vi "Roller Loop.vi"   [LabVIEW 2015]
uses:
  Common Code/Roller Indicators.ctl
  Common Code/Roller Mode Enum.ctl
  Common Code/Auto Roller Commands.ctl
  Common Code/Inner Roller States.ctl
  Sensors/Pot Data.ctl
  Untip Can States.ctl
  Roller Modes.ctl
  Really Real Manual Align.ctl
  Common Code/Change Detect Int.vi
  Robot Global Data.vi
  <vilib>/Rock Robotics/WPI/Solenoid/Deprecated/WPI_SolenoidSetBool.vi
types:
  T1 = typedef "Roller Modes.ctl" = cluster{"Auto Roller Command":T2, "Roller Mode":T3, "Override Intake Speed":dbl}
  T2 = typedef "Auto Roller Commands.ctl" = enum16{"Drag Tote", "Grab Tote", "Idle", "Eject Tote", "Untip Can", "Grab Can"}
  T3 = typedef "Roller Mode Enum.ctl" = enum16{"Manual", "Safe", "Auto"}
  T4 = typedef "Inner Roller States.ctl" = enum16{"Turn Tote Portrait", "Acquire Tote", "Absorb Tote", "Turn Tote Right", "Turn Tote Left", "Acquire Can", "Absorb Can", "Turn Can", "Hold Tote"}
  T5 = typedef "Roller Indicators.ctl" = cluster{"Rollers Closed?":bool, "Roller Mode":T3, "Auto Roller State":T2, "Tote Inside?":bool, "Intake State":T4, "Left Ping Dist":sgl, "Right Ping Dist":sgl, "Potentiometer Cluster":T6, "PING Decision":T4, "Left Arm Closed?":bool, "Portrait?":bool, "Right Arm Closed?":bool, "Left Out":sgl, "Right Out":sgl, "Left Current":sgl, "Right Current":sgl, "Tote Load Complete?":bool, "Untip Complete?":bool, "Untip State":T7, "Roller Safety Open":bool}
  T6 = typedef "Pot Data.ctl" = cluster{"Left Pot Zero":sgl, "Right Pot Zero":sgl, "Left Potentiometer":sgl, "Right Potentiometer":sgl, "Left Pot Non Zero":sgl, "Right Pot Non Zero":sgl}
  T7 = typedef "Untip Can States.ctl" = enum16{"Release Can", "Catch Can", "Idle"}
  T8 = typedef "Dashboard Control Data.ctl" = cluster{"Cam Exposure":dbl, "Go to angle":dbl, "Steer PID Gains":cluster{"proportional gain (Kc)":dbl, "integral time (Ti, min)":dbl, "derivative time (Td, min)":dbl}, "Steer PID output Range":cluster{"output high":dbl, "output low":dbl}, "Pressure m \nValue":dbl, "Pressure b \nValue":dbl, "Roller Command Cluster ":T9, "Elevator":T10, "Encoder Control":T12, "Auton Settings":cluster{"Drive Dist Window Size":dbl}, "Drivetrain Settings":T13, "Lance":T14}
  T9 = typedef "Roller Control.ctl" = cluster{"Intake Speed":dbl, "Turn In Speed":dbl, "Unload Speed":dbl, "Turn Out Speed":dbl, "Ping Align Tolerance":dbl, "Tote Range Threshold":dbl, "Right Pot 0":dbl, "Pot Threshold":dbl, "Left Pot 0":dbl, "Right Pot Scale":dbl, "Left Pot Scale":dbl, "Min Elevator Height":dbl, "Eject Time":dbl, "Eject US Threshold":dbl, "Anti-Twitch Time":u32, "Ping Caring Threshold":dbl, "Pot Diff Threshold":dbl, "Pinch Sustain":u32, "Absorb Give Up Threshold":dbl, "Untip In Threshold":dbl, "Untip Grab Range":dbl, "Ultrasonic Hold Time":u32, "Landscape Absorb Time":u32, "Pot Use Wait Time":u32, "Can Turn Stop Range":dbl, "HP Load Speed":dbl, "Stick Multiplier":dbl, "Coop Eject Speed":dbl}
  T10 = typedef "Elevator DB Control.ctl" = cluster{"PID Output Range":cluster{"output high":dbl, "output low":dbl}, "PID gains":cluster{"proportional gain (Kc)":dbl, "integral time (Ti, min)":dbl, "derivative time (Td, min)":dbl}, "Height Tolerance":sgl, " Encoder Constant":dbl, "Eject Time":sgl, "Zeroing Speed":sgl, "Presets":T11, "Ping Detect Threshold":sgl, "Trashcan Detect Threshold":sgl, "Zero Filter Time":dbl, "Stabilizer Open Time":dbl, "Zero Creep Speed":dbl, "Max Current":dbl, "Current Trip Time":dbl, "Abort Pitch":dbl, "Finger m":dbl, "Finger b":dbl, "Finger max ":dbl, "Finger Stabilizer":dbl, "Finger Store":dbl, "Finger Stop Store":dbl, "Stabilizer Close Time":dbl, "Finger min":dbl, "Unstick gain":dbl, "Full Detect Max":dbl}
  T11 = typedef "Elevator Presets.ctl" = cluster{"Pickup 2 w/ Tote":sgl, "Pickup 2 w/ Trashcan":sgl, "Pickup 3 w/ Tote":sgl, "Pickup 3 w/ Trashcan":sgl, "Bottom":sgl, "Pickup 1 w/ Tote":sgl, "Pickup Trashcan":sgl, "Pickup 1 w/ Trashcan":sgl, "Eject":sgl, "Hold Low":sgl, "Step add height":sgl, "Untip Lift":dbl, "Drop Stack":dbl, "HP Load Hold":dbl, "HP Load Drop":dbl, "HP Load Hold Can":dbl, "Store can max":dbl, "HP Drag Score":dbl, "HP Drag Finish":dbl, "Finger trashcan avoid":dbl, "Full":dbl}
  T12 = typedef "Encoder Control.ctl" = cluster{"Left Tick Constant":dbl, "Right Tick Constant":dbl, "Center Tick Constant":dbl, "Reset?":bool, "Y Dist":cluster{"PID gains":cluster{"proportional gain (Kc)":dbl, "integral time (Ti, min)":dbl, "derivative time (Td, min)":dbl}}, "X Dist":cluster{"PID gains":cluster{"proportional gain (Kc)":dbl, "integral time (Ti, min)":dbl, "derivative time (Td, min)":dbl}}, "Y Stop Thresh":dbl, "Y Stop Speed":dbl, "X Stop Thresh":dbl, "X Stop Speed":dbl}
  T13 = typedef "Drivetrain Settings.ctl" = cluster{"Gyro Tolerance":sgl, "Strafe Correct max steer":sgl, "Strafe Timer Wait":sgl, "Throttle Ramp (ms)":sgl, "Strafe Ramp (ms)":sgl, "Angular rate compensation":bool, "Throttle to Rate Scale":sgl, "Rate compensation gain":sgl, "Creep Steer":sgl, "Creep Throttle":sgl}
  T14 = typedef "Pike DB Controls.ctl" = cluster{"Down Speed":dbl, "Up Speed":dbl, "Max Down Time":dbl, "Max Up Time":dbl, "Current Limit":dbl}
  T15 = typedef "Ultrasonic Indicators.ctl" = cluster{"Left Distance":dbl, "Right Distance":dbl, "Center Distance":dbl, "Left Distance Unfilter":dbl, "Right Distance Unfilter":dbl, "Center Distance Unfilter":dbl}
  T16 = typedef "Roller Manual Bools.ctl" = cluster{"Manual Claw":bool, "Manual Align":T17, "Left Speed":dbl, "Right Speed":dbl}
  T17 = typedef "Really Real Manual Align.ctl" = enum16{"In", "Left", "Right", "Out", "Idle", "HP Load", "Speeds"}
  T18 = typedef "Elevator Status.ctl" = cluster{"Height":dbl, "Enc Value":dbl, "Limit Override":bool, "Mode":T19, "High IR":bool, "Motor Out":dbl, "Ping Detect":bool, "Auto Elevator Indicators":T20, "Master Current":dbl, "Slave Current":dbl, "High Current":bool, "Current Tripped":bool, "Top Limit":bool, "Bottom Limit":bool, "Eject Piston":bool, "Stabilizer":bool, "Finger":bool, "Finger Height":dbl, "Finger Raw":dbl, "Finger at Bottom":bool}
  T19 = typedef "Elevator Mode.ctl" = enum16{"Manual", "Safe", "Auto"}
  T20 = typedef "Auto Elevator Indicators.ctl" = cluster{"Target Out":dbl, "Storing Trashcan?":bool, "State":T21, "In Range":bool, "Store Can Command":bool, "HP Load":bool}
  T21 = typedef "Elevator State.ctl" = enum16{"Idle", "Goto Load Position", "Wait for Load", "Load Drop", "Load Lift", "Drop Stack", "Goto Eject Position", "Eject ", "Raise Trashcan", "Open Stabilizer", "Untip Drop", "Untip Wait", "Untip Lift", "Abort Load", "HP Load Wait", "HP Load Drop", "HP Load Lift", "HP Load Abort", "Close Stabilizer", "HP Load Unfinish", "HP Load Score", "HP Load Finish", "HP Goto Finish Down", "HP Goto Finish Up", "Full"}
  T22 = typedef "WPI_MotorControlDeviceRef.ctl" = cluster{"DeviceStatus":errorcluster, "Type":T23, "PWM":cluster{"PWM Channel":T24, "DeadBand":T25}, "CAN":cluster{"Device Number":u8, "Control Mode":T26, "Semaphore":T27, "Max Vout":dbl, "TalonSRX Control Mode":T28}, "Invert":bool, "TransformRef":T29, "InvTransformRef":T29}
  T23 = typedef "WPI_MotorControlType.ctl" = enum16{"PWM", "CAN", "CANTalonSRX"}
  T24 = typedef "FPGA_DIOPWMChannel.ctl" = enum8{"PWM 0", "PWM 1", "PWM 2", "PWM 3", "PWM 4", "PWM 5", "PWM 6", "PWM 7", "PWM 8", "PWM 9", "PWM MXP 0", "PWM MXP 1", "PWM MXP 2", "PWM MXP 3", "PWM MXP 4", "PWM MXP 5", "PWM MXP 6", "PWM MXP 7", "PWM MXP 8", "PWM MXP 9", "Invalid"}
  T25 = typedef "WPI_PWMDeadband.ctl" = cluster{"Name":string, "maxPositivePwm":i32, "minPositivePwm":i32, "centerPwm":i32, "maxNegativePwm":i32, "minNegativePwm":i32, "angularRange":u16}
  T26 = typedef "WPI_CANJaguar_ControlMode.ctl" = enum8{"Percent VBus", "Current", "Speed", "Position", "Voltage"}
  T27 = typedef "Semaphore RefNum" = refnum<k1>
  T28 = typedef "WPI_CANTalonSRX_APIControlMode.ctl" = enum8{"Percent VBus", "Speed", "Position", "Slave", "Unchanged / Invalid"}
  T29 = typedef "WPI_PWMTransform_ConPane.ctl" = refnum<vi>
  T30 = typedef "WPI_SolenoidDevRef.ctl" = cluster{"DevStatus":errorcluster, "Pneumatics Control Module":u8, "Forward Solenoid Channel":T31, "Reverse Solenoid Channel":T31}
  T31 = typedef "WPI_SolenoidChannel.ctl" = enum8{"Solenoid 0", "Solenoid 1", "Solenoid 2", "Solenoid 3", "Solenoid 4", "Solenoid 5", "Solenoid 6", "Solenoid 7", "Invalid"}
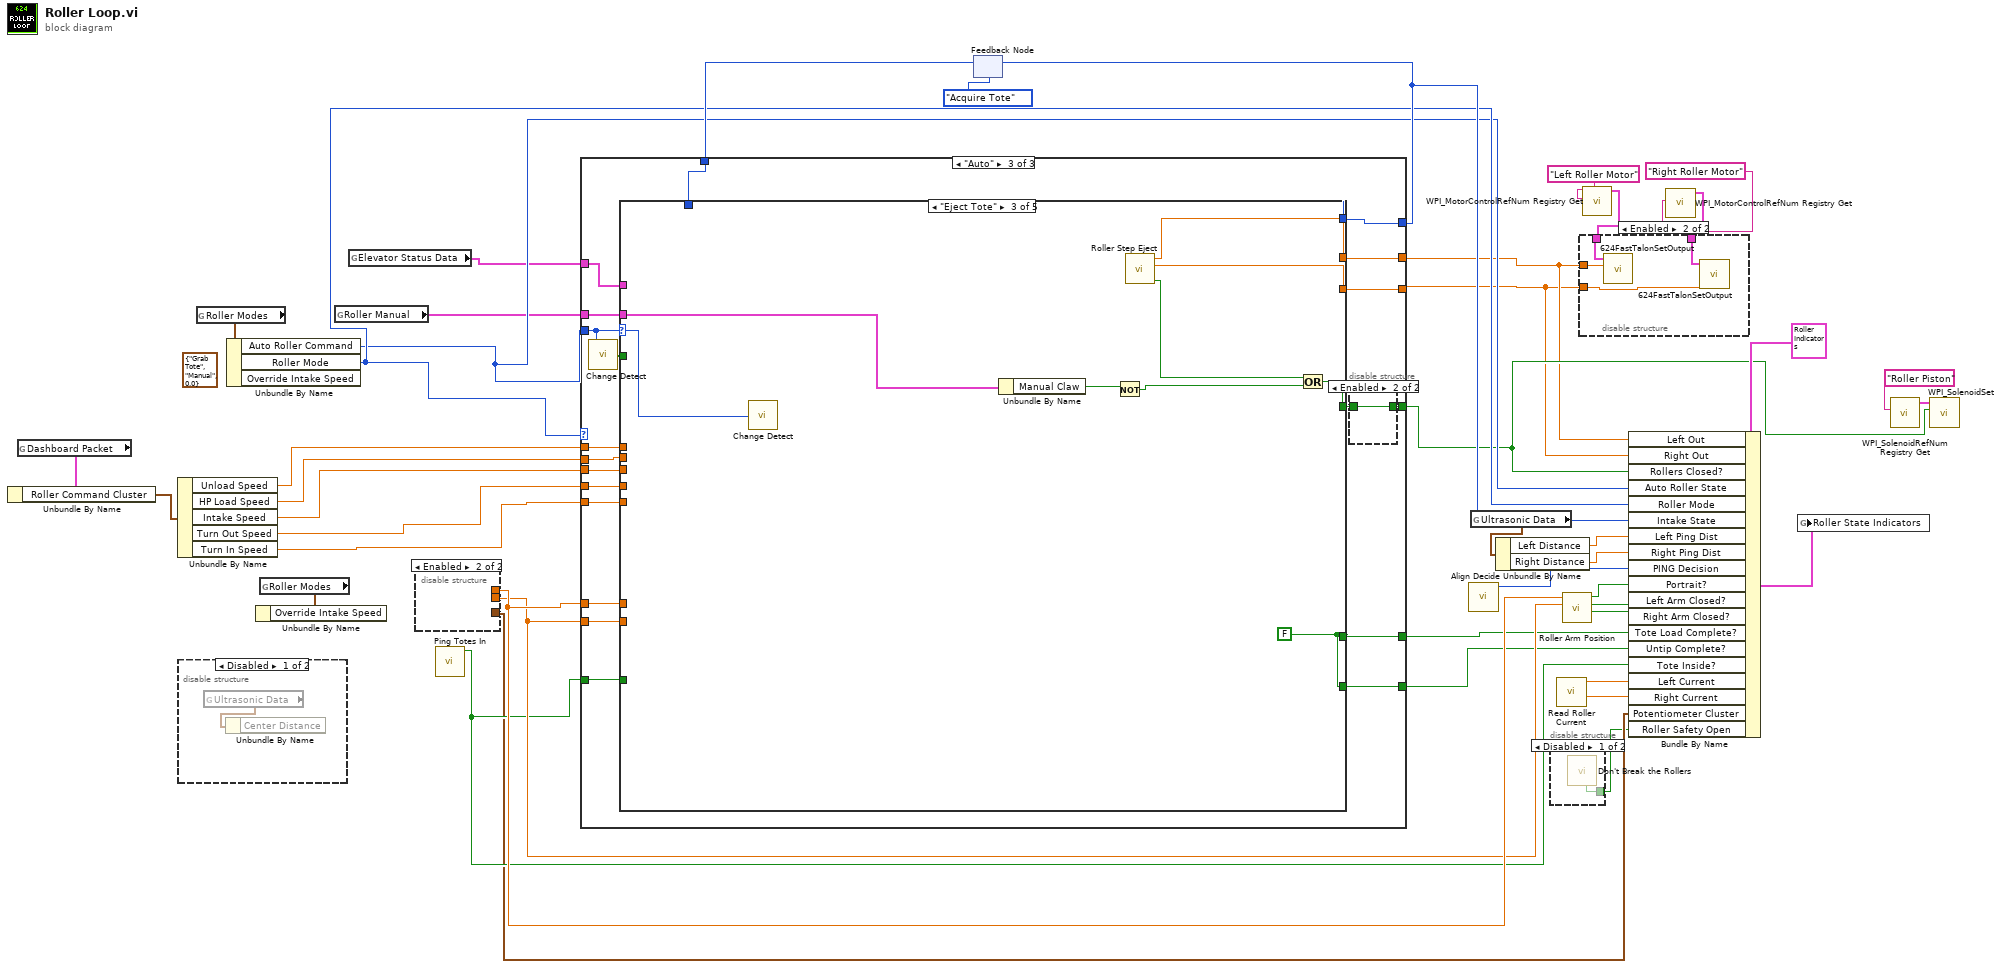
[diagram p0: block diagram]
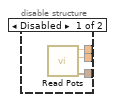
[diagram p2: hidden frame]
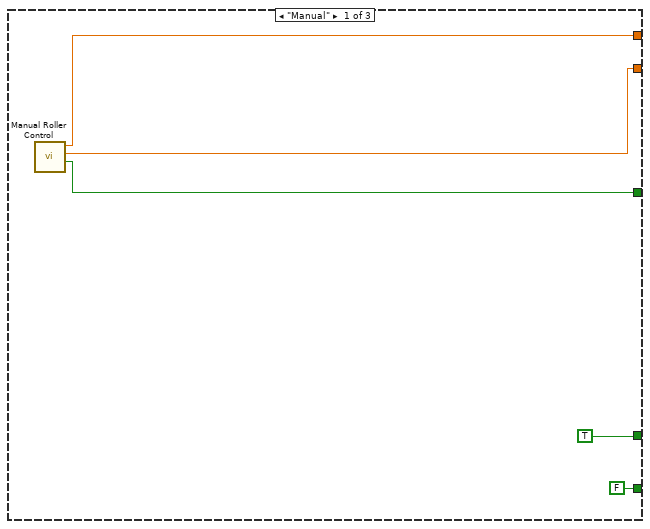
[diagram p4: hidden frame]
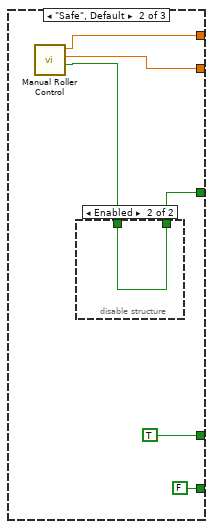
[diagram p5: hidden frame]
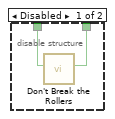
[diagram p6: hidden frame]
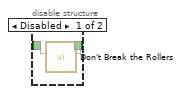
[diagram p7: hidden frame]
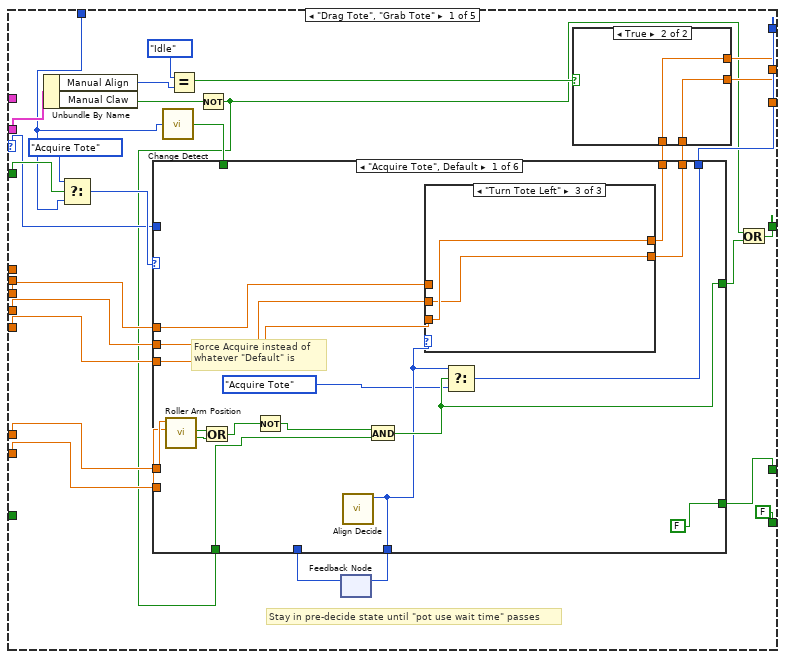
[diagram p8: hidden frame]
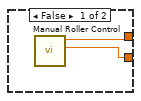
[diagram p9: hidden frame]
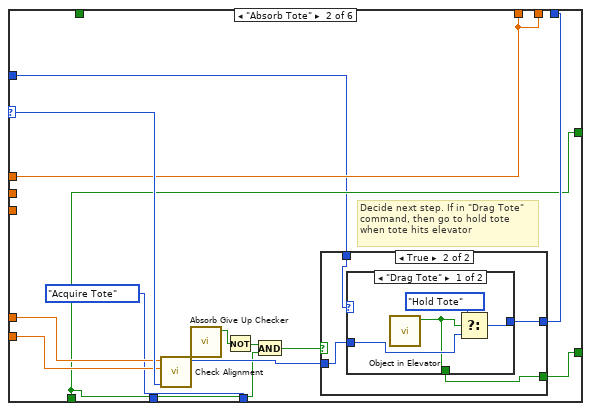
[diagram p12: hidden frame]
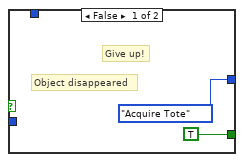
[diagram p13: hidden frame]
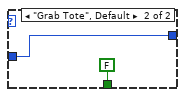
[diagram p14: hidden frame]
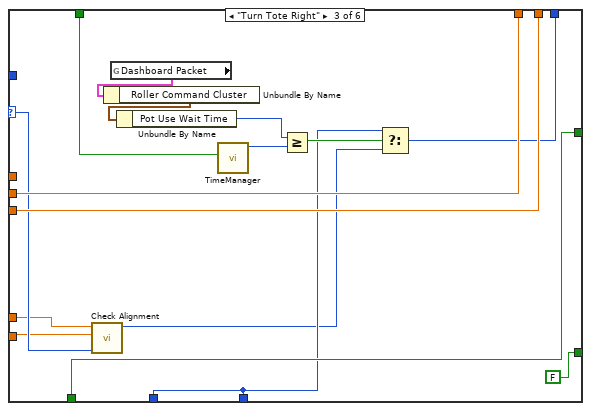
[diagram p15: hidden frame]
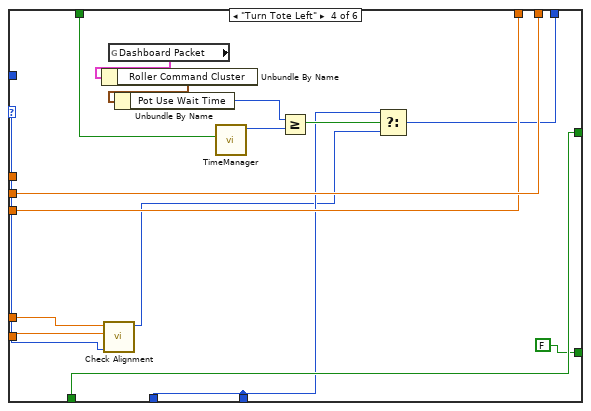
[diagram p16: hidden frame]
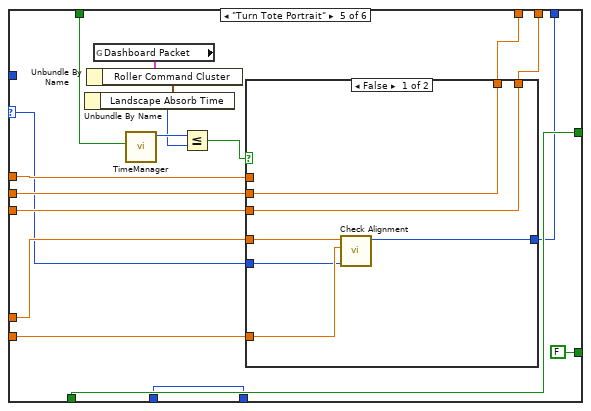
[diagram p17: hidden frame]
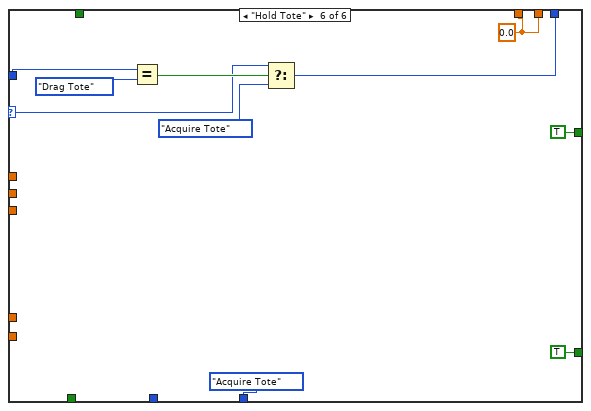
[diagram p19: hidden frame]
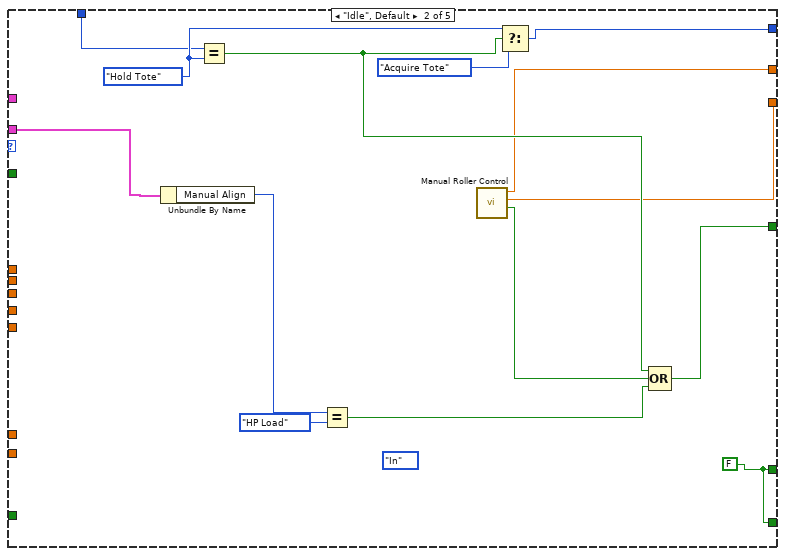
[diagram p20: hidden frame]
diagram:
  (unwired) T1 {"Auto Roller Command"=enum."Grab Tote", "Roller Mode"=enum."Manual", "Override Intake Speed"=0.0} ("input cluster")
  n1 = global read "Robot Global Data.vi" "Dashboard Packet"() -> (w24:T8)
  n2 = Unbundle By Name(w24) -> ("Roller Command Cluster"=w25:T9)
  n3 = Unbundle By Name(w25) -> ("Unload Speed"=w12:dbl, "HP Load Speed"=w4:dbl, "Intake Speed"=w11:dbl, "Turn Out Speed"=w2:dbl, "Turn In Speed"=w1:dbl)
  n4 = disable-structure shown="Disabled" {
    frame Disabled {
      n5 = global read "Robot Global Data.vi" "Ultrasonic Data"() -> (w44:T15)
      n6 = Unbundle By Name(w44) -> ()  [unwired: 1 out]
    }
    frame Enabled {
    }
  }
  n7 = global read "Robot Global Data.vi" "Roller Modes"() -> (w38:T1)
  n8 = Unbundle By Name(w38) -> ("Auto Roller Command"=w35:T2, "Roller Mode"=w36:T3)  [unwired: 1 out]
  n9 = global read "Robot Global Data.vi" "Roller Modes"() -> (w3:T1)
  n10 = Unbundle By Name(w3) -> ()  [unwired: 1 out]
  n11 = global read "Robot Global Data.vi" "Roller Manual"() -> (w20:T16)
  n12 = global read "Robot Global Data.vi" "Elevator Status Data"() -> (w21:T18)
  n13 = disable-structure shown="Enabled" {
    disable-tunnel: [w47 _] -> w29
    disable-tunnel: [w46 _] -> w28
    disable-tunnel: [w45 _] -> w7
    frame Disabled {
      n14 = call "Read Pots.vi"() -> ("Pot Write Cluster"=w45:T6, "Right Pot"=w46:dbl, "Left Pot"=w47:dbl)  [unwired: 7 in, 2 out]
    }
    frame Enabled {
    }
  }
  n15 = call "Ping Totes In.vi"() -> ("In?"=w10:bool)  [unwired: 11 in]
  n16 = feedback #1(Inner_Roller_States."Acquire Tote" ("Enum")) -> (w42:T4)
  n17 = case shown="\"Auto\"" w36 {
    tunnel: w20 -> [_ _ w72]
    tunnel: w11 -> [_ _ w80]
    tunnel: w2 -> [_ _ w78]
    tunnel: w1 -> [_ _ w79]
    tunnel: w35 -> [_ _ w63]
    tunnel: [_ _ w76] -> w37
    tunnel: w42 -> [_ _ w81]
    tunnel: [w48 w58 w69] -> w33
    tunnel: w10 -> [_ _ w77]
    tunnel: [w50 w55 w75] -> w27
    tunnel: [w49 w54 w74] -> w26
    tunnel: w12 -> [_ _ w73]
    tunnel: w29 -> [_ _ w71]
    tunnel: w28 -> [_ _ w70]
    tunnel: [TRUE TRUE w67] -> w23
    tunnel: w21 -> [_ _ w66]
    tunnel: [FALSE FALSE w64] -> w22
    tunnel: w4 -> [_ _ w62]
    frame "Manual" {
      n18 = call "Manual Roller Control.vi"() -> ("Boolean"=w48:bool, "Right Speed Out"=w49:dbl, "Left Speed Out"=w50:dbl)  [unwired: 9 in]
    }
    frame "Safe", Default {
      n19 = call "Manual Roller Control.vi"() -> ("Boolean"=w53:bool, "Right Speed Out"=w54:dbl, "Left Speed Out"=w55:dbl)  [unwired: 9 in]
      n20 = disable-structure shown="Enabled" {
        disable-tunnel: [w60 w61] -> w58
        disable-tunnel: w53 -> [w59 w61]
        frame Disabled {
          n21 = call "Don't Break the Rollers.vi"("Rollers close in"=w59) -> ("Roller close out"=w60:bool)  [unwired: 9 in, 1 out]
        }
        frame Enabled {
        }
      }
    }
    frame "Auto" {
      n22 = call-poly "Change Detect.vi"("In"=w63) -> ("Changed?"=w65:bool)
      n23 = case shown="\"Eject Tote\"" w63 {
        selector: w63 -> [w88 _ w253 _ _]
        tunnel: w81 -> [w91 w240 w255 w270 w323]
        tunnel: [w87 w241 w250 w260 w305] -> w68
        tunnel: w80 -> [w112 _ _ w268 w319]
        tunnel: w79 -> [w111 _ _ _ w317]
        tunnel: w78 -> [w110 _ _ _ w318]
        tunnel: w77 -> [_ _ _ _ _]
        tunnel: [w100 w239 w255 w270 w314] -> w76
        tunnel: [w99 w234 w252 w263 w315] -> w75
        tunnel: [w96 w233 w251 w263 w316] -> w74
        tunnel: w73 -> [_ _ _ _ _]
        tunnel: w72 -> [w106 w245 w247 w257 w325]
        tunnel: w71 -> [w109 _ _ _ _]
        tunnel: w70 -> [w108 _ _ _ _]
        tunnel: [w107 w244 w254 FALSE FALSE] -> w67
        tunnel: w66 -> [_ _ _ w271 _]
        tunnel: w65 -> [w92 _ _ w267 w324]
        tunnel: [FALSE w244 w254 w262 FALSE] -> w64
        tunnel: w62 -> [_ _ _ _ _]
        frame "Drag Tote", "Grab Tote" {
          # "Stay in pre-decide state until \"pot use wait time\" passes"
          n24 = Unbundle By Name(w106) -> ("Manual Align"=w103:T17, "Manual Claw"=w105:bool)
          n25 = Select(t=Inner_Roller_States."Acquire Tote", s=w92, f=w91) -> (s? t:f=w89:T4)
          n26 = call-poly "Change Detect.vi"("In"=w91) -> ("Changed?"=w95:bool)
          n27 = Equal?(x=Really_Real_Manual_Align."Idle" ("y"), y=w103) -> (x = y?=w101:bool)
          n28 = Not(x=w105) -> (.not. x?=w85:bool)
          n29 = feedback #2() -> (w93:T4)  [unwired: 1 in]
          n30 = case shown="\"Acquire Tote\", Default" w89 {
            selector: w89 -> [_ w149 w177 w195 w201 w224]
            tunnel: w85 -> [w123 w143 w174 w190 w207 _]
            tunnel: [w122 w143 w174 w190 w207 TRUE] -> w86
            tunnel: [w133 w151 w164 w182 w200 w222] -> w100
            tunnel: w112 -> [w132 w146 _ _ w210 _]
            tunnel: w111 -> [w131 _ w179 w191 w204 _]
            tunnel: w110 -> [w130 _ w178 w192 w205 _]
            tunnel: [w129 w146 w178 w191 w209 w231] -> w98
            tunnel: [w128 w146 w179 w192 w208 w231] -> w97
            tunnel: w109 -> [w127 w148 w176 w194 w202 _]
            tunnel: w108 -> [w126 w147 w175 w193 w203 _]
            tunnel: [FALSE w145 FALSE FALSE FALSE TRUE ("Boolean")] -> w107
            tunnel: w95 -> [_ _ w170 w185 w213 _]
            tunnel: [w118 Inner_Roller_States."Acquire Tote" ("Next Step") w166 w184 w196 Inner_Roller_States."Acquire Tote" ("Next Step")] -> w94
            tunnel: w93 -> [_ _ w166 w184 w196 _]
            tunnel: w88 -> [_ w139 _ _ _ w227]
            frame "Acquire Tote", Default {
              # "Force Acquire instead of \nwhatever \"Default\" is"
              n31 = call "Roller Arm Position.vi"("Right Pot"=w126, "Left Pot"=w127) -> ("Right Closed?"=w125:bool, "Left Closed?"=w124:bool)  [unwired: 6 in, 2 out]
              n32 = Or(x=w124, y=w125) -> (x .or. y?=w121:bool)
              n33 = Not(x=w121) -> (.not. x?=w120:bool)
              n34 = call "Align Decide.vi"() -> ("Next Step"=w118:T4)  [unwired: 11 in]
              n35 = And(x=w120, y=w123) -> (x .and. y?=w122:bool)
              n36 = case shown="\"Turn Tote Left\"" w118 {
                tunnel: w132 -> [w134 _ _]
                tunnel: w131 -> [_ w136 w138]
                tunnel: w130 -> [_ w135 w137]
                tunnel: [w134 w135 w138] -> w129
                tunnel: [w134 w136 w137] -> w128
                frame "Absorb Tote", Default {
                }
                frame "Turn Tote Right" {
                }
                frame "Turn Tote Left" {
                }
              }
              n37 = Select(t=w118, s=w122, f=Inner_Roller_States."Acquire Tote") -> (s? t:f=w133:T4)
            }
            frame "Absorb Tote" {
              # "Decide next step. If in \"Drag Tote\"\ncommand, then go to hold tote\nwhen tote hits elevator"
              n38 = call "Check Alignment.vi"("Current State"=w149, "Right Pot"=w147, "Left Pot"=w148) -> ("State Output"=w150:T4)  [unwired: 8 in]
              n39 = call "Absorb Give Up Checker.vi"() -> ("Give Up?"=w144:bool)  [unwired: 11 in]
              n40 = Not(x=w144) -> (.not. x?=w142:bool)
              n41 = And(x=w142, y=w143) -> (x .and. y?=w141:bool)
              n42 = case shown="True" w141 {
                tunnel: [Inner_Roller_States."Acquire Tote" ("State Output") w155] -> w151
                tunnel: w150 -> [_ w156]
                tunnel: [TRUE w154] -> w145
                tunnel: w139 -> [_ w157]
                frame False {
                  # "Object disappeared"
                  # "Give up!"
                }
                frame True {
                  n43 = case shown="\"Drag Tote\"" w157 {
                    tunnel: w156 -> [w161 w163]
                    tunnel: [w160 w163] -> w155
                    tunnel: [w158 FALSE ("Boolean")] -> w154
                    frame "Drag Tote" {
                      n44 = call "Object in Elevator.vi"() -> ("Ping Detect"=w158:bool)  [unwired: 11 in]
                      n45 = Select(t=Inner_Roller_States."Hold Tote", s=w158, f=w161) -> (s? t:f=w160:T4)
                    }
                    frame "Grab Tote", Default {
                    }
                  }
                }
              }
            }
            frame "Turn Tote Right" {
              n46 = call "Check Alignment.vi"("Current State"=w177, "Right Pot"=w175, "Left Pot"=w176) -> ("State Output"=w165:T4)  [unwired: 8 in]
              n47 = global read "Robot Global Data.vi" "Dashboard Packet"() -> (w172:T8)
              n48 = Unbundle By Name(w172) -> ("Roller Command Cluster"=w171:T9)
              n49 = Unbundle By Name(w171) -> ("Pot Use Wait Time"=w168:u32)
              n50 = call "TimeManager.vi"("Reset?"=w170) -> ("Time Since Reset"=w169:u32)  [unwired: 9 in, 1 out]
              n51 = Greater Or Equal?(x=w168, y=w169) -> (x >= y?=w167:bool)
              n52 = Select(t=w166, s=w167, f=w165) -> (s? t:f=w164:T4)
            }
            frame "Turn Tote Left" {
              n53 = call "Check Alignment.vi"("Current State"=w195, "Right Pot"=w193, "Left Pot"=w194) -> ("State Output"=w183:T4)  [unwired: 8 in]
              n54 = global read "Robot Global Data.vi" "Dashboard Packet"() -> (w180:T8)
              n55 = Unbundle By Name(w180) -> ("Roller Command Cluster"=w181:T9)
              n56 = Unbundle By Name(w181) -> ("Pot Use Wait Time"=w187:u32)
              n57 = call "TimeManager.vi"("Reset?"=w185) -> ("Time Since Reset"=w186:u32)  [unwired: 9 in, 1 out]
              n58 = Greater Or Equal?(x=w187, y=w186) -> (x >= y?=w188:bool)
              n59 = Select(t=w184, s=w188, f=w183) -> (s? t:f=w182:T4)
            }
            frame "Turn Tote Portrait" {
              n60 = global read "Robot Global Data.vi" "Dashboard Packet"() -> (w199:T8)
              n61 = Unbundle By Name(w199) -> ("Roller Command Cluster"=w198:T9)
              n62 = Unbundle By Name(w198) -> ("Landscape Absorb Time"=w197:u32)
              n63 = call "TimeManager.vi"("Reset?"=w213) -> ("Time Since Reset"=w212:u32)  [unwired: 9 in, 1 out]
              n64 = Less Or Equal?(x=w212, y=w197) -> (x <= y?=w211:bool)
              n65 = case shown="False" w211 {
                tunnel: [w219 w221] -> w209
                tunnel: w210 -> [_ w221]
                tunnel: [w218 w221] -> w208
                tunnel: w205 -> [w219 _]
                tunnel: w204 -> [w218 _]
                tunnel: w203 -> [w217 _]
                tunnel: w202 -> [w216 _]
                tunnel: w201 -> [w215 w220]
                tunnel: [w214 w220] -> w200
                frame False {
                  n66 = call "Check Alignment.vi"("Current State"=w215, "Right Pot"=w217, "Left Pot"=w216) -> ("State Output"=w214:T4)  [unwired: 8 in]
                }
                frame True {
                }
              }
            }
            frame "Hold Tote" {
              w231 = 0.0
              n67 = Equal?(x=w227, y=Auto_Roller_Commands."Drag Tote") -> (x = y?=w225:bool)
              n68 = Select(t=w224, s=w225, f=Inner_Roller_States."Acquire Tote") -> (s? t:f=w222:T4)
            }
          }
          n69 = feedback-in #2(w94) -> ()
          n70 = case shown="True" w101 {
            tunnel: [w114 w116] -> w99
            tunnel: w98 -> [_ w116]
            tunnel: [w113 w115] -> w96
            tunnel: w97 -> [_ w115]
            frame False {
              n71 = call "Manual Roller Control.vi"() -> ("Right Speed Out"=w113:dbl, "Left Speed Out"=w114:dbl)  [unwired: 9 in, 1 out]
            }
            frame True {
            }
          }
          n72 = Or(x=w85, y=w86) -> (x .or. y?=w87:bool)
        }
        frame "Idle", Default {
          (unwired) Really_Real_Manual_Align."In" ("Manual Align")
          w243 = Inner_Roller_States."Hold Tote" ("y")
          w244 = FALSE
          n73 = Unbundle By Name(w245) -> ("Manual Align"=w237:T17)
          n74 = Equal?(x=w240, y=w243) -> (x = y?=w242:bool)
          n75 = Equal?(x=w237, y=Really_Real_Manual_Align."HP Load") -> (x = y?=w235:bool)
          n76 = call "Manual Roller Control.vi"() -> ("Boolean"=w232:bool, "Right Speed Out"=w233:dbl, "Left Speed Out"=w234:dbl)  [unwired: 9 in]
          n77 = Select(t=w243, s=w242, f=Inner_Roller_States."Acquire Tote") -> (s? t:f=w239:T4)
          n78 = Compound Arithmetic op=OR(w242, w232, w235) -> (w241:bool)
        }
        frame "Eject Tote" {
          w254 = FALSE
          n79 = call-poly "Change Detect.vi"("In"=w253) -> ()  [unwired: 1 out]
          n80 = Unbundle By Name(w247) -> ("Manual Claw"=w248:bool)
          n81 = Not(x=w248) -> (.not. x?=w249:bool)
          n82 = call "Roller Step Eject.vi"() -> ("Close Rollers?"=w246:bool, "Right Out"=w251:dbl, "Left Out"=w252:dbl)  [unwired: 9 in]
          n83 = Or(x=w246, y=w249) -> (x .or. y?=w250:bool)
        }
        frame "Untip Can" {
          n84 = feedback #3(Untip_Can_States."Idle") -> (w266:T7)
          n85 = Select(t=Untip_Can_States."Idle", s=w267, f=w266) -> (s? t:f=w265:T7)
          n86 = case shown="\"Release Can\"" w265 {
            selector: w265 -> [w273 w284 w298]
            tunnel: w271 -> [_ _ w294]
            tunnel: w268 -> [_ w287 w301]
            tunnel: [0.0 ("Intake Speed") w287 w301] -> w263
            tunnel: [FALSE TRUE FALSE] -> w256
            tunnel: [TRUE FALSE FALSE] -> w262
            tunnel: [w273 w283 w297] -> w261
            frame "Release Can" {
            }
            frame "Catch Can" {
              n87 = global read "Robot Global Data.vi" "Dashboard Packet"() -> (w280:T8)
              n88 = global read "Robot Global Data.vi" "Ultrasonic Data"() -> (w278:T15)
              n89 = Unbundle By Name(w278) -> ("Center Distance"=w279:dbl)
              n90 = Unbundle By Name(w280) -> ("Roller Command Cluster.Untip In Threshold"=w281:dbl)
              n91 = Less Or Equal?(x=w279, y=w281) -> (x <= y?=w282:bool)
              n92 = Select(t=Untip_Can_States."Release Can", s=w282, f=w284) -> (s? t:f=w283:T7)
            }
            frame "Idle", Default {
              n93 = global read "Robot Global Data.vi" "Dashboard Packet"() -> (w289:T8)
              n94 = global read "Robot Global Data.vi" "Ultrasonic Data"() -> (w291:T15)
              n95 = Unbundle By Name(w289) -> ("Roller Command Cluster.Untip Grab Range"=w290:dbl)
              n96 = Unbundle By Name(w291) -> ("Center Distance"=w292:dbl)
              n97 = Unbundle By Name(w294) -> ("Auto Elevator Indicators.In Range"=w295:bool)
              n98 = Less Or Equal?(x=w292, y=w290) -> (x <= y?=w293:bool)
              n99 = And(x=w295, y=w293) -> (x .and. y?=w296:bool)
              n100 = Select(t=Untip_Can_States."Catch Can", s=w296, f=w298) -> (s? t:f=w297:T7)
            }
          }
          n101 = feedback-in #3(w261) -> ()
          n102 = Unbundle By Name(w257) -> ("Manual Claw"=w258:bool)
          n103 = Not(x=w258) -> (.not. x?=w259:bool)
          n104 = Or(x=w259, y=w256) -> (x .or. y?=w260:bool)
        }
        frame "Grab Can" {
          n105 = Unbundle By Name(w325) -> ("Manual Align"=w320:T17, "Manual Claw"=w302:bool)
          n106 = global read "Robot Global Data.vi" "Dashboard Packet"() -> (w309:T8)
          n107 = global read "Robot Global Data.vi" "Ultrasonic Data"() -> (w310:T15)
          n108 = Unbundle By Name(w310) -> ("Center Distance"=w308:dbl)
          n109 = Unbundle By Name(w309) -> ("Roller Command Cluster.Can Turn Stop Range"=w307:dbl)
          n110 = Not(x=w302) -> (.not. x?=w303:bool)
          n111 = Select(t=Inner_Roller_States."Acquire Can", s=w324, f=w323) -> (s? t:f=w321:T4)
          n112 = Less Or Equal?(x=w308, y=w307) -> (x <= y?=w306:bool)
          n113 = Or(x=w303, y=w306) -> (x .or. y?=w313:bool)
          n114 = case shown="\"Absorb Can\"" w321 {
            selector: w321 -> [w328 w334 w343]
            tunnel: w320 -> [_ _ w344]
            tunnel: [w330 w335 w339] -> w315
            tunnel: w319 -> [w330 w335 w337]
            tunnel: w318 -> [_ _ w340]
            tunnel: w317 -> [_ _ w338]
            tunnel: [w330 w335 w341] -> w316
            tunnel: [w327 w332 w342] -> w314
            tunnel: w313 -> [w329 w331 _]
            tunnel: [w329 w331 TRUE] -> w304
            frame "Absorb Can" {
              n115 = Select(t=w328, s=w329, f=Inner_Roller_States."Acquire Can") -> (s? t:f=w327:T4)
            }
            frame "Acquire Can", Default {
              n116 = Select(t=Inner_Roller_States."Turn Can", s=w331, f=w334) -> (s? t:f=w332:T4)
            }
            frame "Turn Can" {
              n117 = case shown="Default" w344 {
                tunnel: w343 -> [_ w349 w352 w353]
                tunnel: [Inner_Roller_States."Absorb Can" ("t") w349 w352 w353] -> w342
                tunnel: [w345 w348 w350 w354] -> w341
                tunnel: w340 -> [_ w348 w351 _]
                tunnel: [w345 w347 w351 w354] -> w339
                tunnel: w338 -> [_ w347 w350 _]
                tunnel: w337 -> [w345 _ _ _]
                frame "In" {
                }
                frame "Left" {
                }
                frame "Right" {
                }
                frame Default {
                  w354 = 0.0
                }
              }
            }
          }
          n118 = Or(x=w304, y=w303) -> (x .or. y?=w305:bool)
        }
      }
      n119 = disable-structure shown="Enabled" {
        disable-tunnel: [w83 w84] -> w69
        disable-tunnel: w68 -> [w82 w84]
        frame Disabled {
          n120 = call "Don't Break the Rollers.vi"("Rollers close in"=w82) -> ("Roller close out"=w83:bool)  [unwired: 9 in, 1 out]
        }
        frame Enabled {
        }
      }
    }
  }
  n121 = feedback-in #1(w37) -> ()
  n122 = call "Align Decide.vi"() -> ("Next Step"=w34:T4)  [unwired: 11 in]
  n123 = global read "Robot Global Data.vi" "Ultrasonic Data"() -> (w13:T15)
  n124 = Unbundle By Name(w13) -> ("Left Distance"=w15:dbl, "Right Distance"=w14:dbl)
  n125 = disable-structure shown="Disabled" {
    disable-tunnel: [w355 _] -> w5
    frame Disabled {
      n126 = call "Don't Break the Rollers.vi"() -> ("Keeep rollers open?"=w355:bool)  [unwired: 10 in, 1 out]
    }
    frame Enabled {
    }
  }
  n127 = call "Read Roller Current.vi"() -> ("R Current"=w8:dbl, "L Current"=w9:dbl)  [unwired: 10 in]
  n128 = call "Roller Arm Position.vi"("Right Pot"=w28, "Left Pot"=w29) -> ("Right Closed?"=w30:bool, "Left Closed?"=w31:bool, "Portrait?"=w32:bool)  [unwired: 6 in, 1 out]
  n129 = call <vilib>:"WPI_MotorControlRefNum Registry Get.vi"("refnum name"="Left Roller Motor") -> ("MotorControlDevRef"=w19:T22)  [unwired: 9 in, 1 out]
  n130 = Bundle By Name(cluster=T5 {"Rollers Closed?"=FALSE, "Roller Mode"=enum."Manual", "Auto Roller State"=enum."Grab Tote", "Tote Inside?"=FALSE, "Intake State"=enum."Acquire Tote", "Left Ping Dist"=0.0, "Right Ping Dist"=0.0, "Potentiometer Cluster"={"Left Pot Zero"=0.0, "Right Pot Zero"=0.0, "Left Potentiometer"=0.0, "Right Potentiometer"=0.0, "Left Pot Non Zero"=0.0, "Right Pot Non Zero"=0.0}, "PING Decision"=enum."Acquire Tote", "Left Arm Closed?"=FALSE, "Portrait?"=FALSE, "Right Arm Closed?"=FALSE, "Left Out"=0.0, "Right Out"=0.0, "Left Current"=0.0, "Right Current"=0.0, "Tote Load Complete?"=FALSE, "Untip Complete?"=FALSE, "Untip State"=enum."Idle", "Roller Safety Open"=FALSE} ("Roller State Indicators"), "Left Out"=w27, "Right Out"=w26, "Rollers Closed?"=w33, "Auto Roller State"=w35, "Roller Mode"=w36, "Intake State"=w37, "Left Ping Dist"=w15, "Right Ping Dist"=w14, "PING Decision"=w34, "Portrait?"=w32, "Left Arm Closed?"=w31, "Right Arm Closed?"=w30, "Tote Load Complete?"=w23, "Untip Complete?"=w22, "Tote Inside?"=w10, "Left Current"=w9, "Right Current"=w8, "Potentiometer Cluster"=w7, "Roller Safety Open"=w5) -> (w41:T5)
  n131 = call <vilib>:"WPI_MotorControlRefNum Registry Get.vi"("refnum name"="Right Roller Motor") -> ("MotorControlDevRef"=w17:T22)  [unwired: 9 in, 1 out]
  n132 = disable-structure shown="Enabled" {
    disable-tunnel: w19 -> [w358 w360]
    disable-tunnel: w27 -> [w359 w363]
    disable-tunnel: w17 -> [w356 w361]
    disable-tunnel: w26 -> [w357 w362]
    frame Disabled {
      n133 = call <vilib>:"WPI_MotorControlSetOutput.vi"("Output"=w359, "MotorControlDevRef"=w358) -> ()  [unwired: 7 in, 3 out]
      n134 = call <vilib>:"WPI_MotorControlSetOutput.vi"("Output"=w357, "MotorControlDevRef"=w356) -> ()  [unwired: 7 in, 3 out]
    }
    frame Enabled {
      n135 = call "624FastTalonSetOutput.vi"("Output"=w363, "MotorControlDevRef"=w360) -> ()  [unwired: 8 in, 2 out]
      n136 = call "624FastTalonSetOutput.vi"("Output"=w362, "MotorControlDevRef"=w361) -> ()  [unwired: 8 in, 2 out]
    }
  }
  n137 = global write "Robot Global Data.vi" "Roller State Indicators"(w41) -> ()
  n138 = call <vilib>:"WPI_SolenoidRefNum Registry Get.vi"("refnum name"="Roller Piston") -> ("SolenoidDevRef"=w39:T30)  [unwired: 9 in, 1 out]
  n139 = call-poly <vilib>:"WPI_SolenoidSet.vi"("Value"=w33, "SolenoidDevRef"=w39) -> ()  [unwired: 8 in, 2 out]
